vi "UDPEngine.Main.vi"(7 "WaveformChart Ref":refnum<vi>, 8 "error in (no error)":errorcluster, 10 "UDP Engine Queue":refnum<queue>, 11 "WorkspaceManager":T1) -> (0 "error out":errorcluster, 1 "Exit":bool, 2 "Update?":bool, 3 "Waveform":waveform(dbl)[](array[waveform]))   [LabVIEW 2015, in "Single Station Execution.lvlib"]
uses:
  Single Station Execution.lvlib
  Types/UDPEngine.QueueCluster.ctl
  Types/UDPEngine.State.ctl
  <vilib>/NI Veristand/Execution/Workspace/WorkspaceAPI.ctl
  NationalInstruments.VeriStand.ClientAPI
  <vilib>/NI Veristand/Execution/Workspace/UDPChannelStreamSession.ctl
  NationalInstruments.VeriStand
  <vilib>/NI Veristand/Execution/Workspace/UDP Stream Packet.ctl
  <vilib>/Utility/tcp.llb/UDP Multicast Read-Only Open.vi
  <vilib>/NI Veristand/Execution/Workspace/NI_VS Workspace ExecutionAPI.lvlib
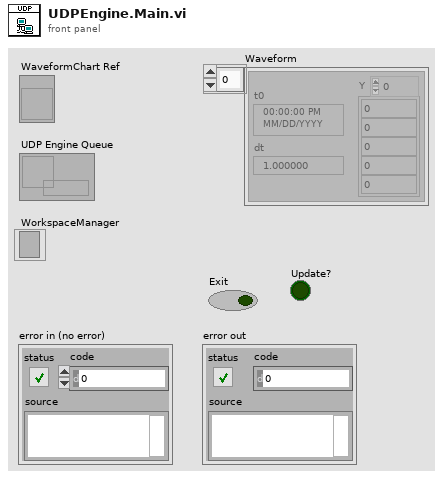
[diagram p1: front panel]
types:
  T1 = typedef "NI_VS Workspace ExecutionAPI.lvlib/WorkspaceAPI.ctl" = refnum<k24>
  T2 = typedef "Single Station Execution.lvlib/UDPEngine.State.ctl" = enum8{"Idle", "Start Acq", "Run", "Stop Acq", "Exit"}
  T3 = typedef "NI_VS Workspace ExecutionAPI.lvlib/UDPChannelStreamSession.ctl" = refnum<k24>
  T4 = cluster{"Initialized Waveform":waveform(dbl)[], "VS UDP Session":T3, "Channel IDs":i32[], "Packet IDs":i32[], "Max Packet Size":i32, "UDP Ref":refnum<k16>}
  T5 = typedef "Single Station Execution.lvlib/UDPEngine.QueueCluster.ctl" = cluster{"Action":T2, "Channels":string[]}
  T6 = typedef "NI_VS Workspace ExecutionAPI.lvlib/UDP Stream Packet.ctl" = cluster{"ID":i32, "t0":dbl, "dt":dbl, "Channel IDs":i32[], "Channel Data":dbl[][], "Sample Offset":u64}
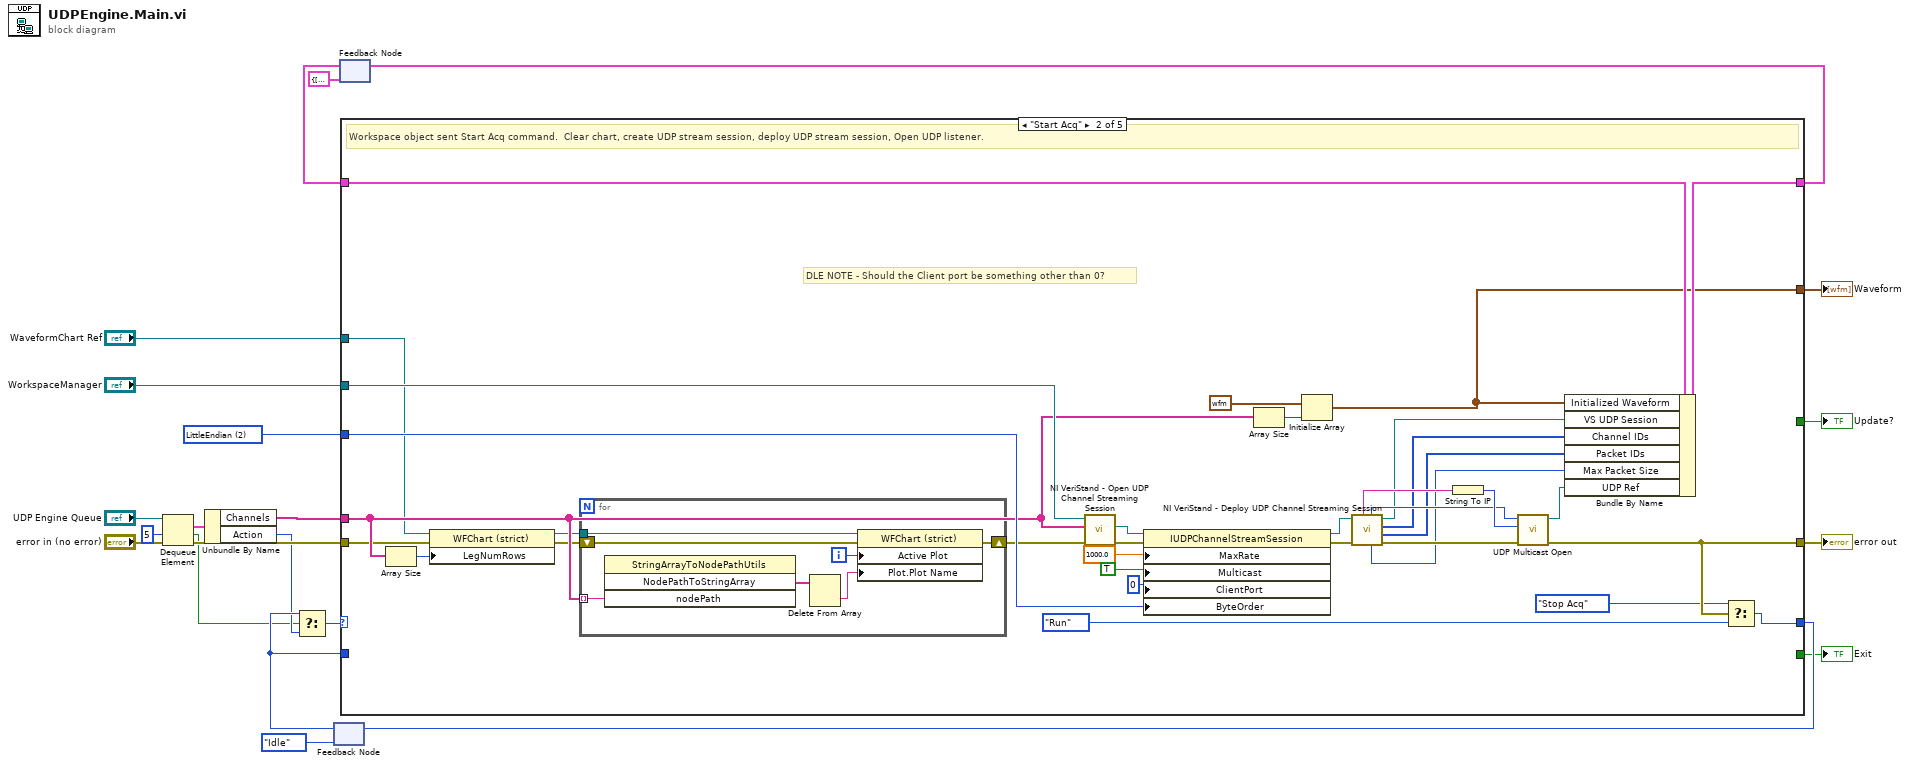
[diagram p0: block diagram]
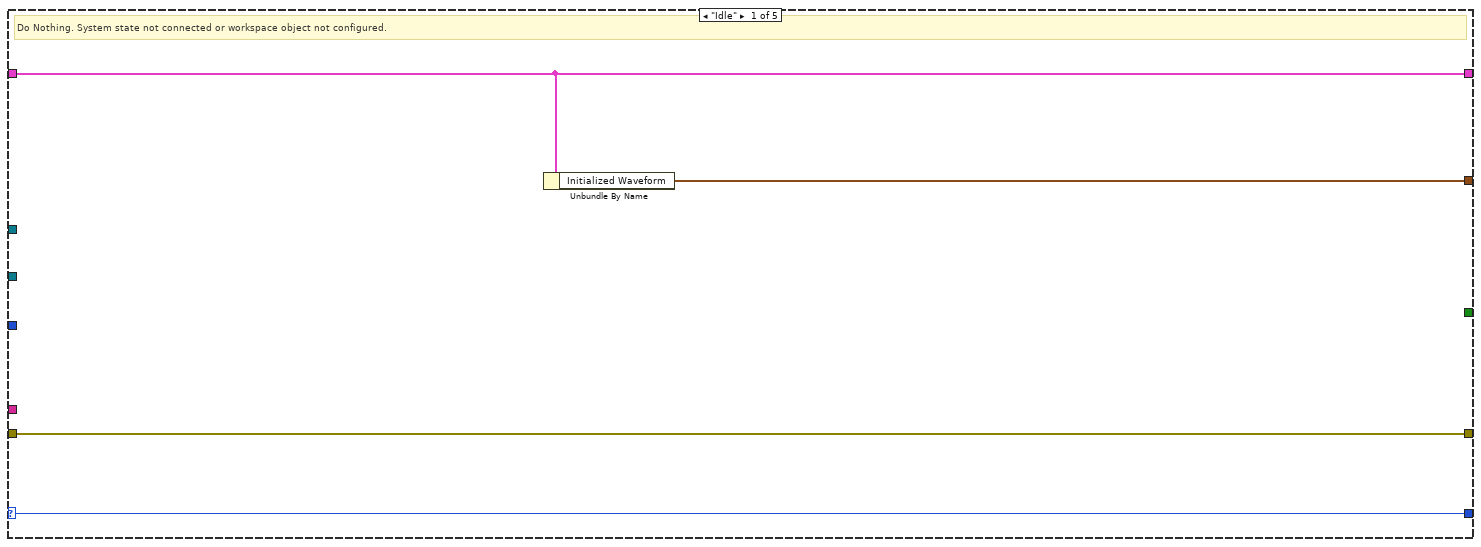
[diagram p2: hidden frame]
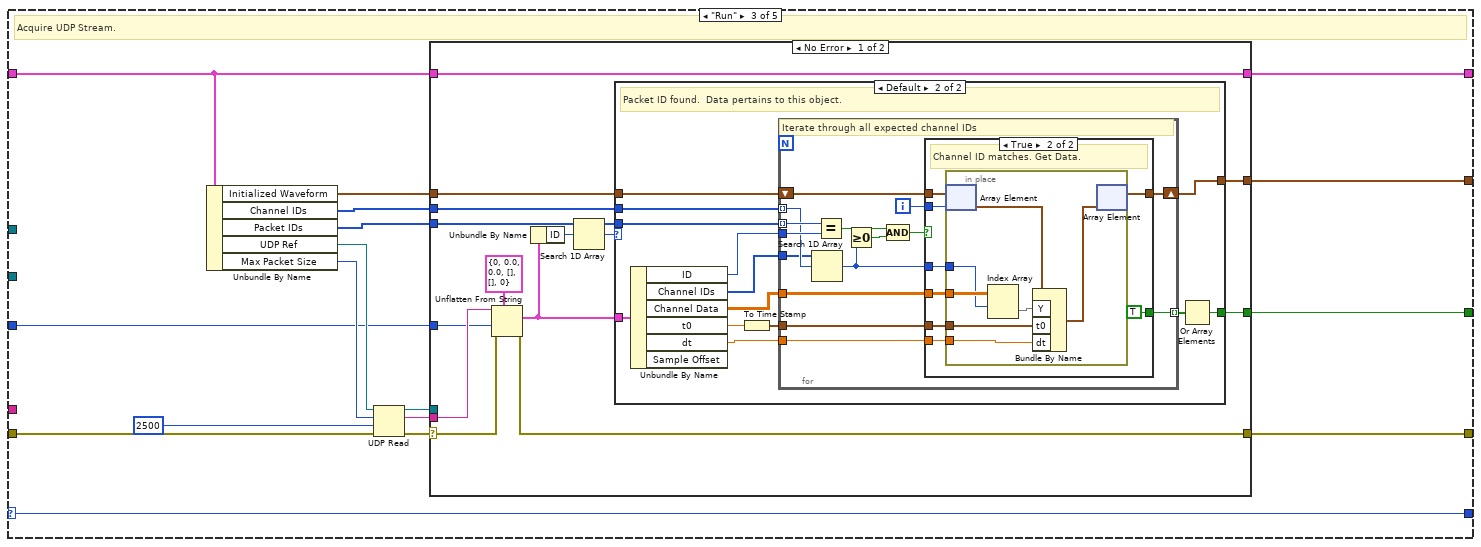
[diagram p3: hidden frame]
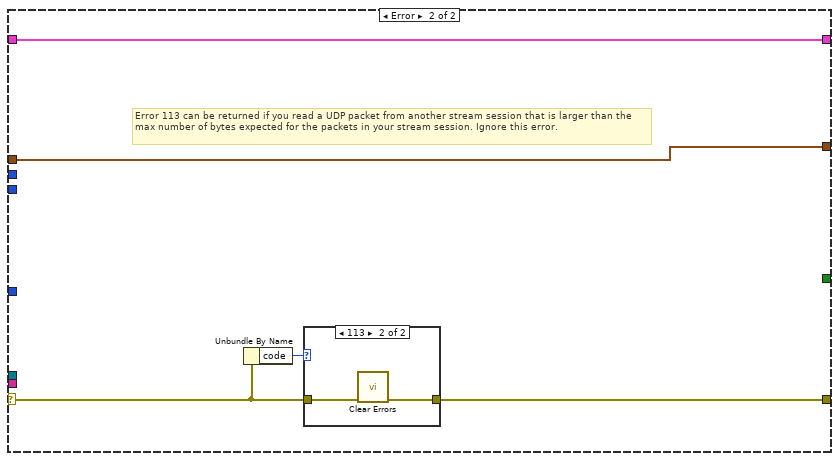
[diagram p6: hidden frame]
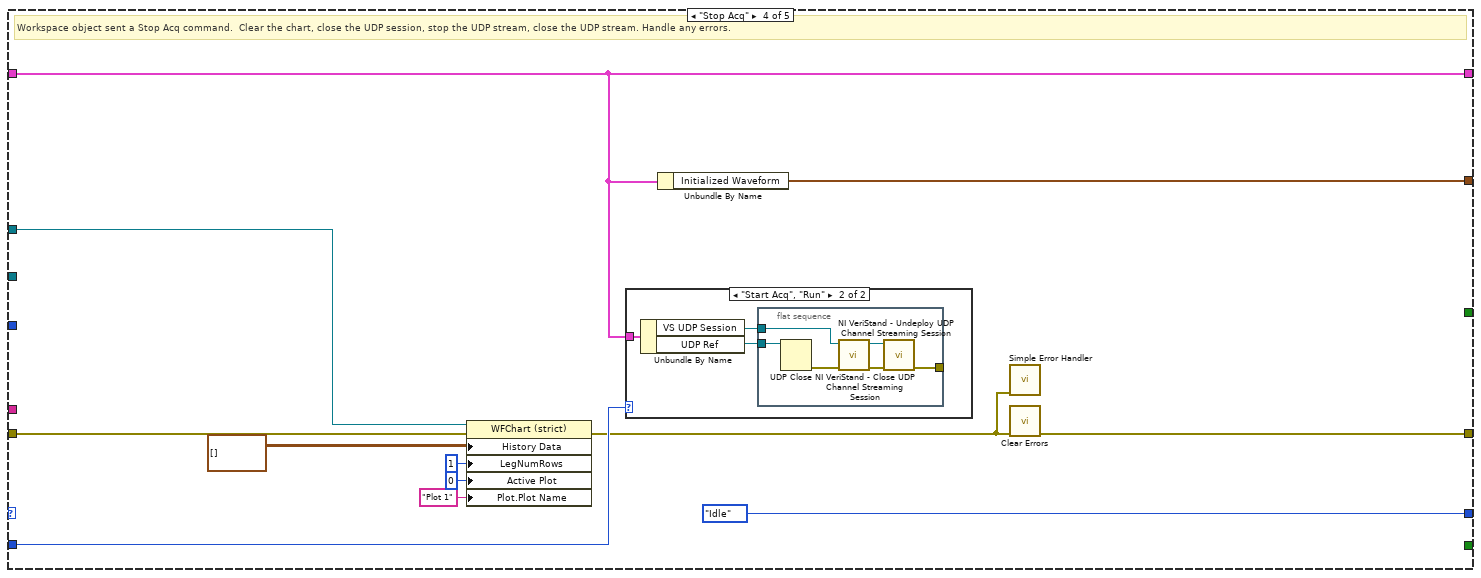
[diagram p8: hidden frame]
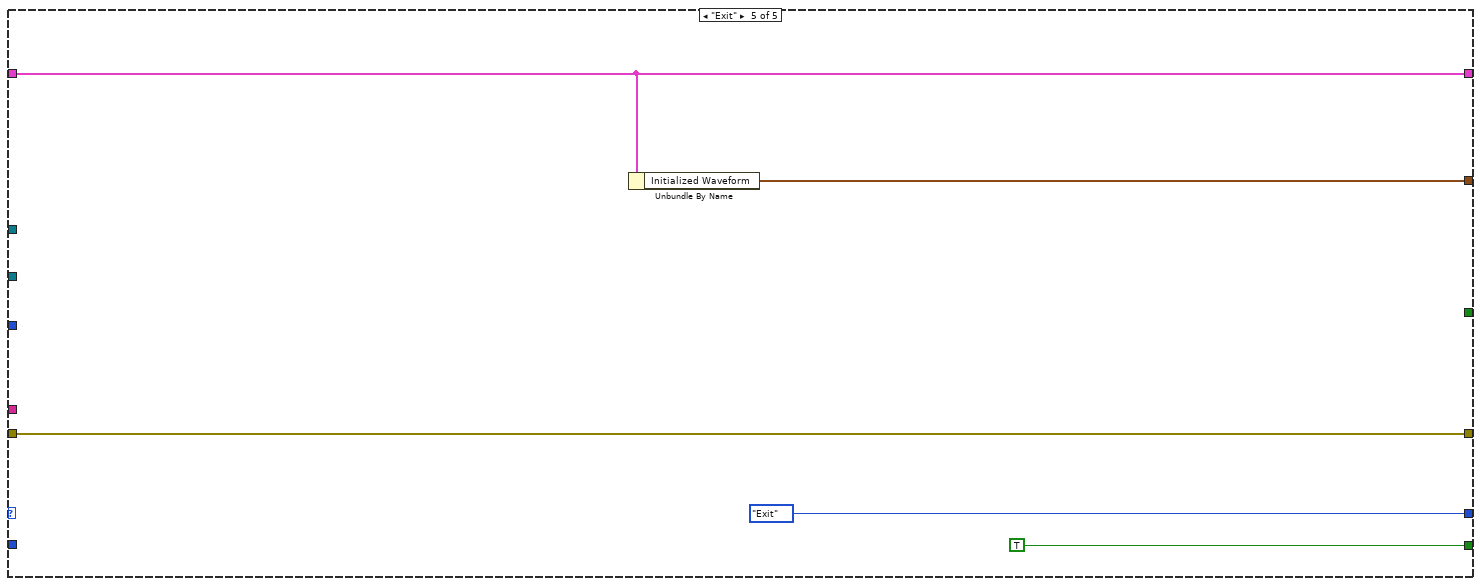
[diagram p10: hidden frame]
diagram:
  w16 = 2 items=["BigEndian", "NativeHostOrder", "LittleEndian"] ("Byte Order")
  n1 = Dequeue Element(queue="UDP Engine Queue", timeout in ms (-1)=5, error in (no error)="error in (no error)") -> (element=w6:T5, timed out?=w8:bool, error out=w12:errorcluster)  [unwired: 1 out]
  n2 = Unbundle By Name(w6) -> ("Channels"=w15:string[], "Action"=w9:T2)
  n3 = feedback #1(UDPEngine.State."Idle" ("Action")) -> (w21:T2)
  n4 = Select(t=w21, s=w8, f=w9) -> (s? t:f=w10:T2)
  n5 = feedback #2(T4 {"Initialized Waveform"=[], "VS UDP Session"=refnum, "Channel IDs"=[], "Packet IDs"=[], "Max Packet Size"=0, "UDP Ref"=refnum}) -> (w18:T4)
  n6 = case shown="\"Start Acq\"" w10 {
    selector: w10 -> [w25 _ w73 _ _]
    tunnel: "WorkspaceManager" -> [_ w48 _ _ _]
    tunnel: w18 -> [w24 w47 w74 w157 w175]
    tunnel: w16 -> [_ w41 w70 _ _]
    tunnel: [w24 w40 w75 w157 w175] -> w17
    tunnel: [w25 w38 w73 UDPEngine.State."Idle" ("Action") UDPEngine.State."Exit" ("Action")] -> w20
    tunnel: [_ _ _ _ TRUE] -> w11
    tunnel: w12 -> [w26 w30 w72 w159 w176]
    tunnel: [w26 w39 w71 w163 w176] -> w13
    tunnel: w15 -> [_ w32 _ _ _]
    tunnel: w21 -> [_ _ _ w162 _]
    tunnel: [w23 w36 w69 w156 w174] -> w22
    tunnel: "WaveformChart Ref" -> [_ w31 _ w161 _]
    tunnel: [_ _ w68 _ _] -> w3
    frame "Idle" {
      # "Do Nothing. System state not connected or workspace object not configured."
      n7 = Unbundle By Name(w24) -> ("Initialized Waveform"=w23:waveform(dbl)[])
    }
    frame "Start Acq" {
      # "DLE NOTE - Should the Client port be something other than 0?"
      # "Workspace object sent Start Acq command.  Clear chart, create UDP stream session, deploy UDP stream session, Open UDP listener."
      n8 = Array Size(array=w32) -> (size(s)=w27:i32)
      n9 = property on="Property Node" class="WFChart (strict)"(reference=w31, error in=w30, "LegNumRows"=w27) -> (reference out=w28:refnum<vi>, error out=w29:errorcluster)
      n10 = for {
        tunnel: w28 -> [w67]
        shift-right: [w65] -> w33
        shift-left: w29 -> [w66]
        tunnel: w32 -> [w63] mode=indexing
        i -> [w64]
        n11 = invoke class="StringArrayToNodePathUtils" method="NodePathToStringArray"("nodePath"=w63) -> ("NodePathToStringArray"=w62:string[])  [unwired: 3 in, 3 out]
        n12 = Delete From Array(array=w62) -> (deleted portion=w61:string)  [unwired: 2 in, 1 out]
        n13 = property on="Property Node" class="WFChart (strict)"(reference=w67, error in=w66, "Active Plot"=w64, "Plot.Plot Name"=w61) -> (error out=w65:errorcluster)  [unwired: 1 out]
      }
      n14 = call <vilib>:"NI VeriStand - Open UDP Channel Streaming Session.vi"("error in (no error)"=w33, "Channels"=w32, "WorkspaceManager in"=w48) -> ("error out"=w58:errorcluster, "UDPChannelStreamSession out"=w55:T3)  [unwired: 6 in, 1 out]
      n15 = property class="IUDPChannelStreamSession"(reference=w55, error in=w58, "MaxRate"=1000.0, "Multicast"=TRUE, "ClientPort"=u16 0, "ByteOrder"=w41) -> (reference out=w57:T3, error out=w56:errorcluster)
      n16 = Array Size(array=w32) -> (size(s)=w53:i32)
      n17 = Initialize Array(waveform(dbl) {"t0"=timestamp(0 s since 1904-01-01), "dt"=1.0, "Y"=[]}, w53) -> (w36:waveform(dbl)[])
      n18 = call <vilib>:"NI VeriStand - Deploy UDP Channel Streaming Session.vi"("error in (no error)"=w56, "UDPChannelStreamSession in"=w57) -> ("error out"=w50:errorcluster, "Packet IDs"=w44:i32[], "Channel IDs"=w45:i32[], "UDPChannelStreamSession out"=w46:T3, "Max Packet Size"=w43:i32, "Port"=w51:u16, "UDP Multicast Address"=w49:string)  [unwired: 3 in]
      n19 = String To IP(1:w49) -> (0:w52:u32)
      n20 = call-poly <vilib>:"UDP Multicast Open.vi"("error in (no error)"=w50, "multicast addr"=w52, "port"=w51) -> ("error out"=w39:errorcluster, "connection ID"=w42:refnum<k16>)  [unwired: 6 in, 1 out]
      n21 = Bundle By Name(cluster=w47, "Initialized Waveform"=w36, "VS UDP Session"=w46, "Channel IDs"=w45, "Packet IDs"=w44, "Max Packet Size"=w43, "UDP Ref"=w42) -> (w40:T4)
      n22 = Select(t=UDPEngine.State."Stop Acq" ("Action"), s=w39, f=UDPEngine.State."Run" ("Action")) -> (s? t:f=w38:T2)
    }
    frame "Run" {
      # "Acquire UDP Stream."
      n23 = Unbundle By Name(w74) -> ("Initialized Waveform"=w80:waveform(dbl)[], "Channel IDs"=w79:i32[], "Packet IDs"=w78:i32[], "UDP Ref"=w77:refnum<k16>, "Max Packet Size"=w76:i32)
      n24 = UDP Read(connection ID=w77, max size (548)=w76, timeout ms (25000)=2500, 8:w72) -> (data out=w82:string, error out=w83:errorcluster, 3:w84:refnum<k16>)  [unwired: 2 out]
      n25 = case shown="No Error" w83 {
        selector: w83 -> [w97 w145]
        tunnel: w78 -> [w92 _]
        tunnel: w82 -> [w95 _]
        tunnel: w79 -> [w94 _]
        tunnel: w80 -> [w93 w146]
        tunnel: [w98 w147] -> w71
        tunnel: w84 -> [_ _]
        tunnel: w70 -> [w88 _]
        tunnel: [w87 w148] -> w75
        tunnel: w74 -> [w87 w148]
        tunnel: [w86 w146] -> w69
        tunnel: [w85 _] -> w68
        frame No Error {
          n26 = Unflatten From String(type=T6 {"ID"=0, "t0"=0.0, "dt"=0.0, "Channel IDs"=[], "Channel Data"=[], "Sample Offset"=0} ("UDP Data Packet"), binary string=w95, byte order (0:big-endian, network order)=w88, error in (no error)=w97) -> (value=w89:T6, error out=w98:errorcluster)  [unwired: 1 in, 1 out]
          n27 = Unbundle By Name(w89) -> ("ID"=w90:i32)
          n28 = Search 1D Array(1D array=w92, element=w90) -> (index of element=w91:i32)  [unwired: 1 in]
          n29 = case shown="Default" w91 {
            tunnel: w94 -> [_ w112]
            tunnel: w93 -> [w99 w111]
            tunnel: w92 -> [_ w109]
            tunnel: w89 -> [_ w108]
            tunnel: [w99 w102] -> w86
            tunnel: [_ w100] -> w85
            frame -1 {
              # "This is a packet from a different UDP session. Ignore it."
            }
            frame Default {
              # "Packet ID found.  Data pertains to this object."
              n30 = Unbundle By Name(w108) -> ("ID"=w107:i32, "Channel IDs"=w106:i32[], "Channel Data"=w105:dbl[][], "t0"=w104:dbl, "dt"=w103:dbl)  [unwired: 1 out]
              n31 = To Time Stamp(1:w104) -> (0:w110:timestamp)
              n32 = for {
                tunnel: w112 -> [w125] mode=indexing
                tunnel: w109 -> [w127] mode=indexing
                tunnel: w107 -> [w126]
                tunnel: w105 -> [w119]
                tunnel: w106 -> [w118]
                shift-right: [w114] -> w102
                shift-left: w111 -> [w117]
                tunnel: w110 -> [w116]
                tunnel: w103 -> [w115]
                tunnel: [w113] -> w101 mode=indexing
                i -> [w120]
                # "Iterate through all expected channel IDs"
                n33 = Search 1D Array(1D array=w118, element=w125) -> (index of element=w121:i32)  [unwired: 1 in]
                n34 = Equal?(x=w127, y=w126) -> (x = y?=w124:bool)
                n35 = Greater Or Equal To 0?(x=w121) -> (x >= 0?=w123:bool)
                n36 = Compound Arithmetic op=AND(w124, w123) -> (w122:bool)
                n37 = case shown="True" w122 {
                  tunnel: w121 -> [_ w134]
                  tunnel: w120 -> [_ w130]
                  tunnel: w119 -> [_ w135]
                  tunnel: w117 -> [w128 w136]
                  tunnel: w116 -> [_ w133]
                  tunnel: w115 -> [_ w132]
                  tunnel: [w128 w131] -> w114
                  tunnel: [_ TRUE] -> w113
                  frame False {
                    # "This channel is not in this UDP Data Packet."
                  }
                  frame True {
                    # "Channel ID matches. Get Data."
                    n38 = in-place {
                      in-place-border: w135 -> [w142]
                      in-place-border: w134 -> [w141]
                      in-place-border: w133 -> [w139]
                      in-place-border: w132 -> [w138]
                      n39 = in-place-array #3(w136, w130) -> (w143:waveform(dbl))
                      n40 = Index Array(array=w142, index (row)=w141) -> (element=w140:dbl[])  [unwired: 1 in]
                      n41 = Bundle By Name(cluster=w143, "Y"=w140, "t0"=w139, "dt"=w138) -> (w137:waveform(dbl))
                      n42 = in-place-array #3(w137) -> (w131:waveform(dbl)[])  [unwired: 1 out]
                    }
                  }
                }
              }
              n43 = Or Array Elements(Boolean array=w101) -> (logical OR=w100:bool)
            }
          }
        }
        frame Error {
          # "Error 113 can be returned if you read a UDP packet from another stream session that is larger than the max number of bytes expected for the packets in your stream session. Ignore this error."
          n44 = Unbundle By Name(w145) -> ("code"=w144:i32)
          n45 = case shown="113" w144 {
            tunnel: [w149 w151] -> w147
            tunnel: w145 -> [w149 w150]
            frame Default {
            }
            frame 113 {
              n46 = call <vilib>:"Clear Errors.vi"("error in (no error)"=w150) -> ("error out"=w151:errorcluster)  [unwired: 5 in, 1 out]
            }
          }
        }
      }
    }
    frame "Stop Acq" {
      # "Workspace object sent a Stop Acq command.  Clear the chart, close the UDP session, stop the UDP stream, close the UDP stream. Handle any errors."
      n47 = property on="Property Node" class="WFChart (strict)"(reference=w161, error in=w159, "History Data"=waveform(dbl)[][] [], "LegNumRows"=u32 1 ("Legend:Number of Rows"), "Active Plot"=u32 0, "Plot.Plot Name"="Plot 1") -> (error out=w158:errorcluster)  [unwired: 1 out]
      n48 = case shown="\"Start Acq\", \"Run\"" w162 {
        tunnel: w157 -> [_ w164]
        frame Default {
        }
        frame "Start Acq", "Run" {
          n49 = Unbundle By Name(w164) -> ("VS UDP Session"=w165:T3, "UDP Ref"=w166:refnum<k16>)
          n50 = flat-sequence {
            tunnel: w166 -> [w169]
            tunnel: w165 -> [w168]
            tunnel: [w167] -> _
            frame #0 {
              n51 = UDP Close(connection ID=w169) -> (error out=w172:errorcluster)  [unwired: 1 in, 1 out]
              n52 = call <vilib>:"NI VeriStand - Undeploy UDP Channel Streaming Session.vi"("error in (no error)"=w172, "UDPChannelStreamSession in"=w168) -> ("error out"=w170:errorcluster, "UDPChannelStreamSession out"=w171:T3)  [unwired: 8 in]
              n53 = call <vilib>:"NI VeriStand - Close UDP Channel Streaming Session.vi"("error in (no error)"=w170, "UDPChannelStreamSession in"=w171) -> ("error out"=w167:errorcluster)  [unwired: 9 in]
            }
          }
        }
      }
      n54 = Unbundle By Name(w157) -> ("Initialized Waveform"=w156:waveform(dbl)[])
      n55 = call <vilib>:"Simple Error Handler.vi"("error in (no error)"=w158) -> ()  [unwired: 4 in, 5 out]
      n56 = call <vilib>:"Clear Errors.vi"("error in (no error)"=w158) -> ("error out"=w163:errorcluster)  [unwired: 5 in, 1 out]
    }
    frame "Exit" {
      n57 = Unbundle By Name(w175) -> ("Initialized Waveform"=w174:waveform(dbl)[])
    }
  }
  "Waveform" <- w22
  "error out" <- w13
  "Exit" <- w11
  "Update?" <- w3
  n58 = feedback-in #1(w20) -> ()
  n59 = feedback-in #2(w17) -> ()
